vi "GetApplicationConfigFile.vi"(8 "error in (no error)":errorcluster) -> (0 "error out":errorcluster, 3 "Application config file Path":path)   [LabVIEW 2011]
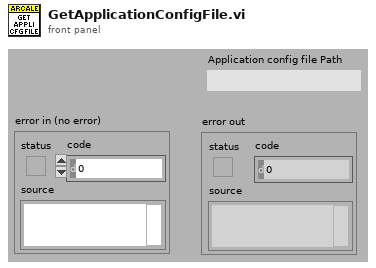
[diagram p1: front panel]
types:
  T1 = typedef "ApplicationInfos.ctl" = cluster{"ApplicationName":string, "ApplicationVersion":string, "Logo 600X200 path":path, "Logo 400X400 path":path, "Client":string}
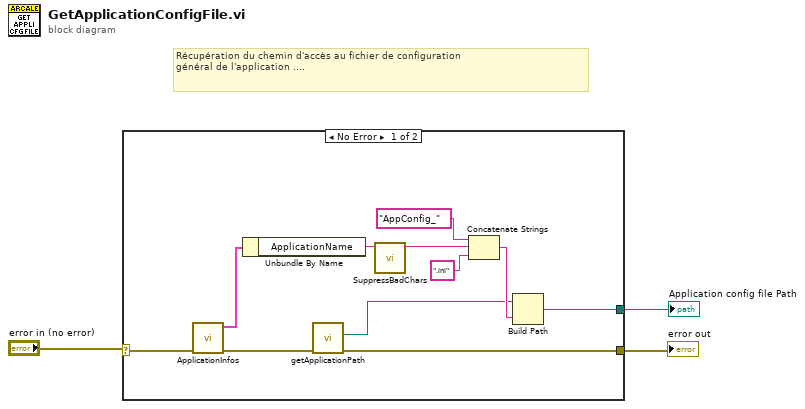
[diagram p0: block diagram]
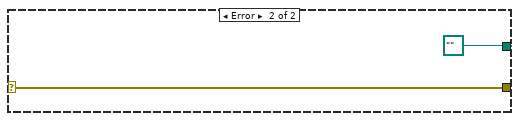
[diagram p2: hidden frame]
diagram:
  # "Récupération du chemin d'accès au fichier de configuration\ngénéral de l'application ...."
  n1 = case shown="No Error" "error in (no error)" {
    selector: "error in (no error)" -> [w14 w16]
    tunnel: [w5 w16] -> w2
    tunnel: [w8 path "" ("Application config file Path")] -> w1
    frame No Error {
      n2 = call "ApplicationInfos.vi"("error in (no error)"=w14) -> ("error out"=w6:errorcluster, "ApplicationInfo"=w13:T1)  [unwired: 9 in]
      n3 = Unbundle By Name(w13) -> ("ApplicationName"=w12:string)
      n4 = call "getApplicationPath.vi"("error in (no error)"=w6) -> ("error out"=w5:errorcluster, "ApplicationPath"=w4:path)  [unwired: 9 in]
      n5 = call "SuppressBadChars.vi"("StringIn"=w12) -> ("StringOut"=w11:string)  [unwired: 9 in, 1 out]
      n6 = Concatenate Strings("AppConfig_" ("string"), w11, ".ini" ("string")) -> (w9:string)
      n7 = Build Path(base path=w4, name or relative path=w9) -> (appended path=w8:path)
    }
    frame Error {
    }
  }
  "error out" <- w2
  "Application config file Path" <- w1
